vi "GUARDAR_DB.vi"(6 "ALARMA":string, 7 "ESTADO TANQUE":string, 8 "error in (no error)":errorcluster, 9 "BOMBA":string, 10 "VELOCIDAD_LLENADO":dbl, 11 "PORCENTAJE_TANQUE":dbl) -> (0 "error out":errorcluster)   [LabVIEW 2019, in "GUARDAR_DATOS_SQL.lvlib"]
doc: "SOLICITAR DATOS PARA GUARDADO EN SQL\n_____\nCreated using Delacor QMH Event Scripter 5.0.0.112."
uses:
  GUARDAR_DATOS_SQL.lvlib
  GUARDAR_DB Argument--cluster.ctl
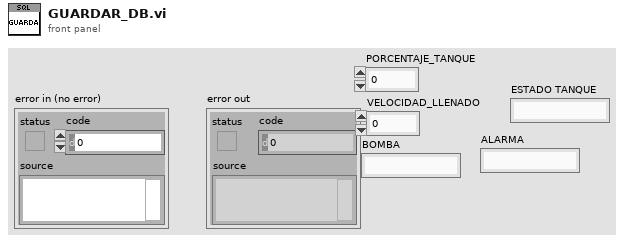
[diagram p1: front panel]
types:
  T1 = typedef "GUARDAR_DATOS_SQL.lvlib/GUARDAR_DB Argument--cluster.ctl" = cluster{"PORCENTAJE_TANQUE":dbl, "VELOCIDAD_LLENADO":dbl, "ESTADO TANQUE":string, "ALARMA":string, "BOMBA":string}
  T2 = typedef "GUARDAR_DATOS_SQL.lvlib/Request Events--cluster.ctl" = cluster{"Stop Module":refnum<user-event>, "Show Panel":refnum<user-event>, "Hide Panel":refnum<user-event>, "Get Module Execution Status":refnum<user-event>, "Show Diagram":refnum<user-event>, "GUARDAR_DB":refnum<user-event>}
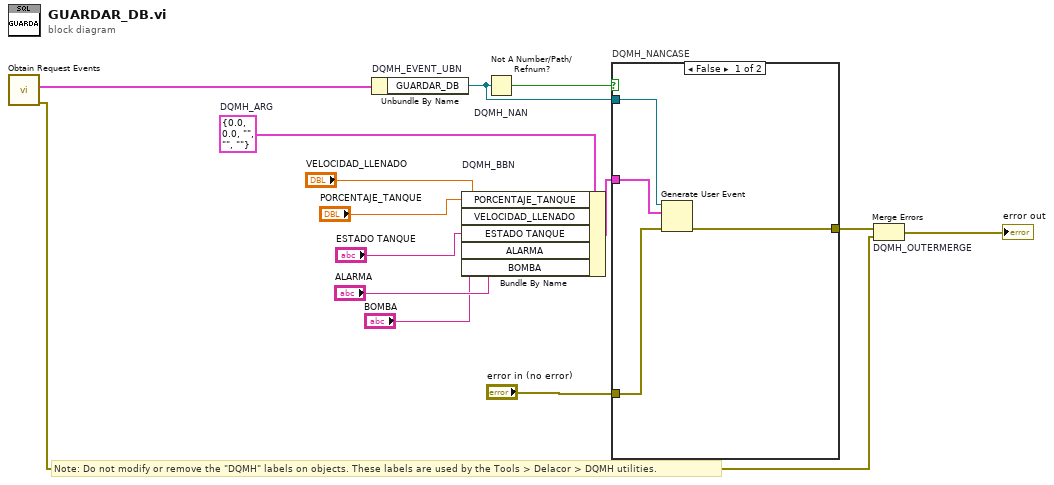
[diagram p0: block diagram]
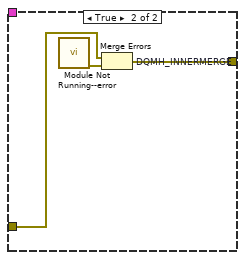
[diagram p2: hidden frame]
diagram:
  w8 = T1 {"PORCENTAJE_TANQUE"=0.0, "VELOCIDAD_LLENADO"=0.0, "ESTADO TANQUE"="", "ALARMA"="", "BOMBA"=""}  # DQMH_ARG
  # "Note: Do not modify or remove the \"DQMH\" labels on objects. These labels are used by the Tools > Delacor > DQMH utilities."
  n1 = call "Obtain Request Events.vi"() -> ("error out"=w7:errorcluster, "GUARDAR_DATOS_SQL Request Events"=w6:T2)  [unwired: 10 in]
  n2 = Unbundle By Name "DQMH_EVENT_UBN"(w6) -> ("GUARDAR_DB"=w10:refnum<user-event>)
  n3 = Bundle By Name "DQMH_BBN"(cluster=w8, "PORCENTAJE_TANQUE"="PORCENTAJE_TANQUE", "VELOCIDAD_LLENADO"="VELOCIDAD_LLENADO", "ESTADO TANQUE"="ESTADO TANQUE", "ALARMA"="ALARMA", "BOMBA"="BOMBA") -> (w12:T1)
  n4 = Not A Number/Path/Refnum? "DQMH_NAN"(number/path/refnum=w10) -> (NaN/Path/Refnum?=w11:bool)
  n5 = case "DQMH_NANCASE" shown="False" w11 {
    tunnel: "error in (no error)" -> [w18 w21]
    tunnel: [w17 w20] -> w9
    tunnel: w10 -> [w16 _]
    tunnel: w12 -> [w15 _]
    frame False {
      n6 = Generate User Event(user event=w16, event data cluster=w15, error in=w18) -> (error out=w17:errorcluster)  [unwired: 1 in, 1 out]
    }
    frame True {
      n7 = call "Module Not Running--error.vi"() -> ("error out"=w19:errorcluster)  [unwired: 11 in]
      n8 = Merge Errors "DQMH_INNERMERGE"(w21, w19) -> (w20:errorcluster)
    }
  }
  n9 = Merge Errors "DQMH_OUTERMERGE"(w9, w7) -> (→"error out":errorcluster)
